vi "fgv_PXIe-2530_visa.vi"(7 "cmd":T1, 8 "error in":errorcluster) -> (0 "error out":errorcluster)   [LabVIEW 2021]
uses:
  ctrl/PXIe-2530_q.ctl
  ctrl/rw.ctl
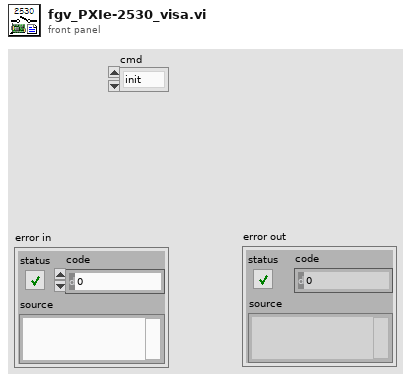
[diagram p1: front panel]
types:
  T1 = typedef "PXIe-2530_q.ctl" = enum16{"init", "write", "close"}
  T2 = typedef "rw.ctl" = enum16{"read", "write"}
  T3 = typedef "PXIe-2530_cfg.ctl" = cluster{"visa":refnum<k15>, "topology":T4, "relay name":string, "relay action":i32}
  T4 = typedef "niSwitch Topologies.ctl" = string
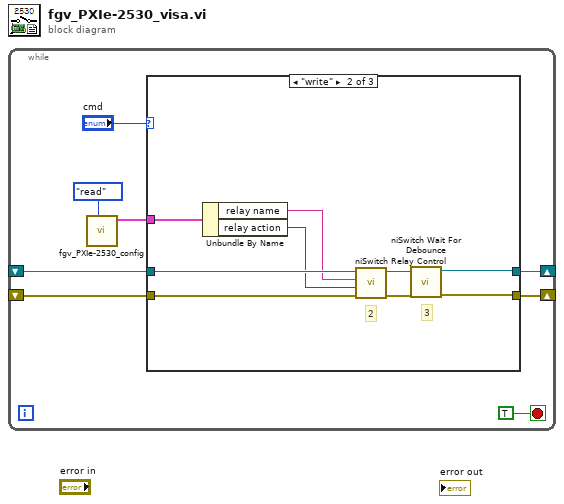
[diagram p0: block diagram]
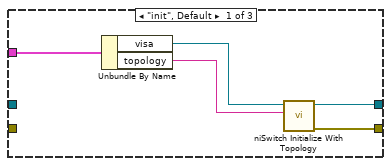
[diagram p2: hidden frame]
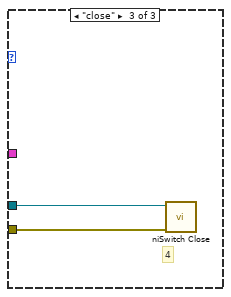
[diagram p3: hidden frame]
diagram:
  n1 = while {
    shift-right: [w5] -> _
    shift-left: _ -> [w6]
    shift-right: [w4] -> _
    shift-left: _ -> [w3]
    stop <- TRUE stop-if-true
    n2 = call "fgv_PXIe-2530_config.vi"("cmd"=rw."read") -> ("config 2"=w1:T3)  [unwired: 10 in]
    n3 = case shown="\"write\"" "cmd" {
      tunnel: w6 -> [_ w19 w23]
      tunnel: [w13 w17 _] -> w5
      tunnel: [w12 w18 _] -> w4
      tunnel: w3 -> [_ w20 w24]
      tunnel: w1 -> [w9 w16 _]
      frame "init", Default {
        n4 = Unbundle By Name(w9) -> ("visa"=w11:refnum<k15>, "topology"=w10:T4)
        n5 = call <instrlib>:"niSwitch Initialize With Topology.vi"("topology name"=w10, "resource name"=w11) -> ("error out"=w13:errorcluster, "instrument handle out"=w12:refnum<k15>)  [unwired: 3 in, 5 out]
      }
      frame "write" {
        # "3"
        # "2"
        n6 = Unbundle By Name(w16) -> ("relay name"=w15:string, "relay action"=w14:i32)
        n7 = call <instrlib>:"niSwitch Relay Control.vi"("error in (no error)"=w19, "relay action (Close Relay)"=w14, "relay names"=w15, "instrument handle"=w20) -> ("error out"=w21:errorcluster, "instrument handle out"=w22:refnum<k15>)  [unwired: 6 out]
        n8 = call <instrlib>:"niSwitch Wait For Debounce.vi"("error in (no error)"=w21, "instrument handle"=w22) -> ("error out"=w17:errorcluster, "instrument handle out"=w18:refnum<k15>)  [unwired: 1 in, 7 out]
      }
      frame "close" {
        # "4"
        n9 = call <instrlib>:"niSwitch Close.vi"("error in (no error)"=w23, "instrument handle"=w24) -> ()  [unwired: 10 out]
      }
    }
  }
